vi "ANAL_SelectSpectrum.vi"(8 "Single Bin Selection":i32(slide) scale=1.0..58.0, 9 "Sweep Selection":i32(slide)=1 min=1 max=58 step=1 scale=1.0..58.0, 10 "Main Data Array":T1 {"Run Data Cluster"."Temperature B" scale=0.0..100.0; "Run Data Cluster"."Temperature A" scale=0.0..100.0}) -> (0 "Selected Spectrum":i32[](array[numeric]), 2 "Main Data Array Out":T1 {"Run Data Cluster"."Temperature B" scale=0.0..100.0; "Run Data Cluster"."Temperature A" scale=0.0..100.0})   [LabVIEW 2021]
uses:
  ANAL_Data.ctl
  XML_Cluster.ctl
  DAT_Cluster.ctl
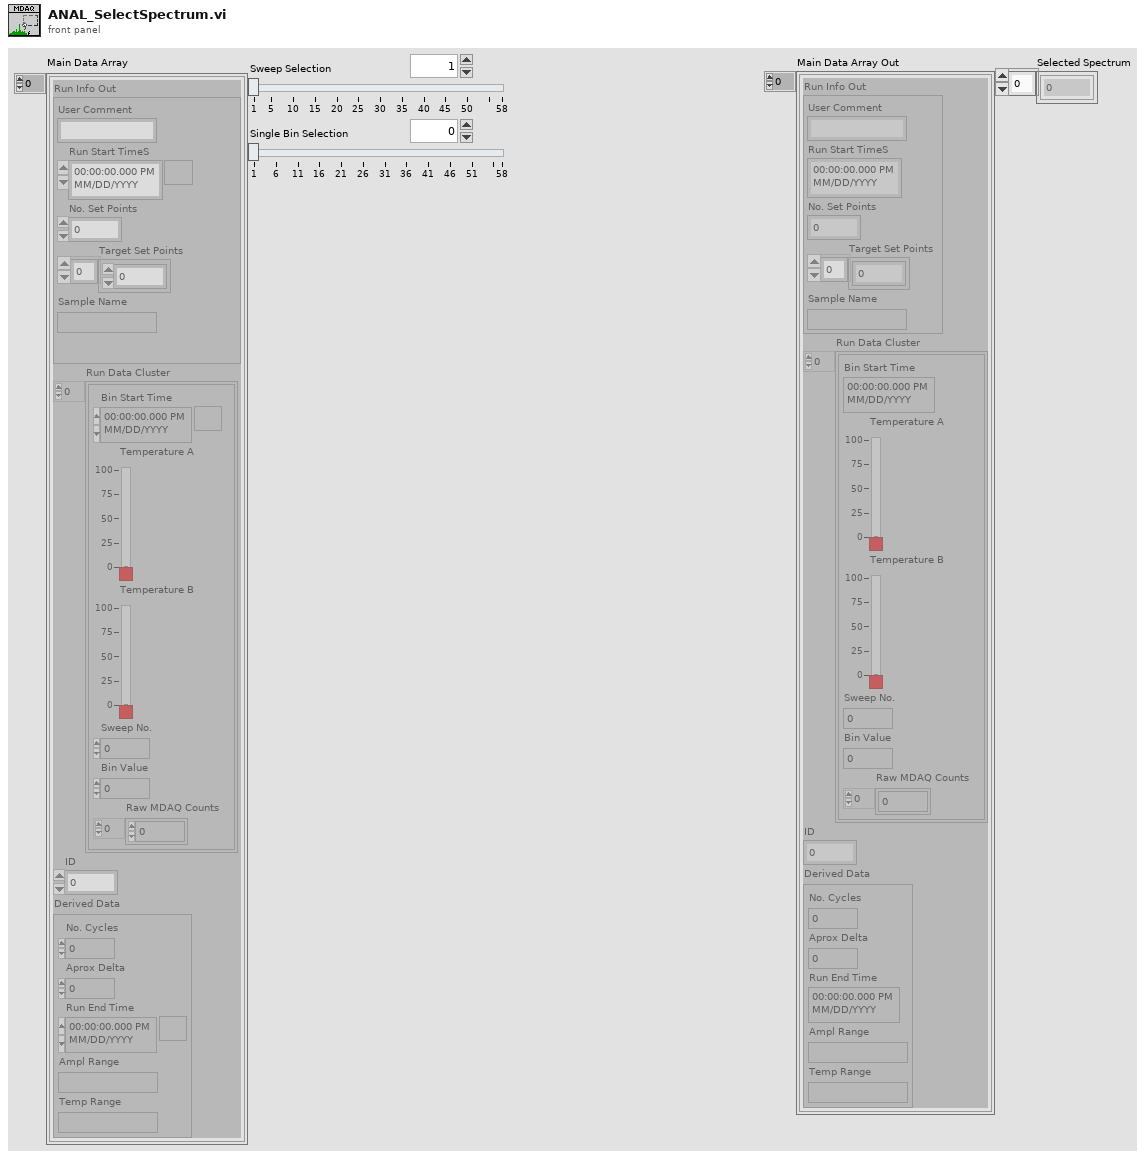
[diagram p1: front panel]
types:
  T1 = typedef "ANAL_Data.ctl" = cluster{"Run Info Out":T2, "Run Data Cluster":T3, "ID":u32, "Derived Data":cluster{"No. Cycles":u32, "Aprox Delta":dbl, "Run End Time":timestamp, "Ampl Range":string, "Temp Range":string}}[]
  T2 = typedef "XML_Cluster.ctl" = cluster{"User Comment":string, "Run Start TimeS":timestamp, "No. Set Points":u32, "Target Set Points":i32[], "Sample Name":string}
  T3 = typedef "DAT_Cluster.ctl" = cluster{"Bin Start Time":timestamp, "Temperature A":dbl, "Temperature B":dbl, "Sweep No.":i32, "Bin Value":i32, "Raw MDAQ Counts":i32[]}[]
  T4 = cluster{"Run Info Out":T2, "Run Data Cluster":T3, "ID":u32, "Derived Data":cluster{"No. Cycles":u32, "Aprox Delta":dbl, "Run End Time":timestamp, "Ampl Range":string, "Temp Range":string}}
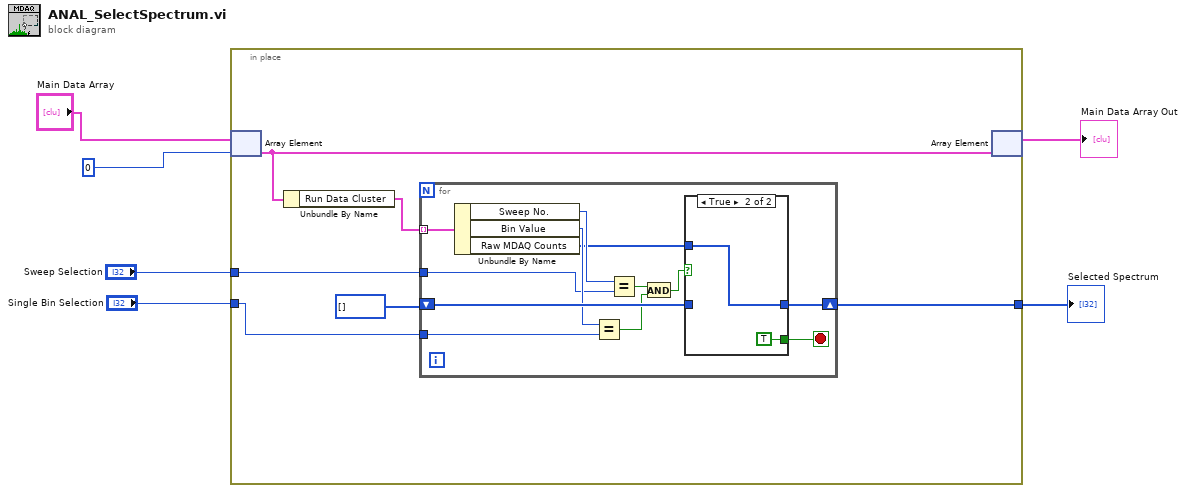
[diagram p0: block diagram]
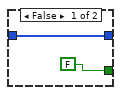
[diagram p2: hidden frame]
diagram:
  n1 = in-place {
    in-place-border: "Sweep Selection" -> [w9]
    in-place-border: "Single Bin Selection" -> [w8]
    in-place-border: [w7] -> w1
    n2 = in-place-array #1("Main Data Array", 0) -> (w12:T4)
    n3 = Unbundle By Name(w12) -> ("Run Data Cluster"=w11:T3)
    n4 = for {
      tunnel: w11 -> [w24] mode=indexing
      shift-right: [w22] -> w7
      shift-left: i32[] [] -> [w23]
      tunnel: w9 -> [w16]
      tunnel: w8 -> [w15]
      stop <- w13 stop-if-true
      n5 = Unbundle By Name(w24) -> ("Sweep No."=w18:i32, "Bin Value"=w17:i32, "Raw MDAQ Counts"=w14:i32[])
      n6 = Equal?(x=w17, y=w15) -> (x = y?=w19:bool)
      n7 = Equal?(x=w18, y=w16) -> (x = y?=w20:bool)
      n8 = And(x=w20, y=w19) -> (x .and. y?=w21:bool)
      n9 = case shown="True" w21 {
        tunnel: w23 -> [w26 _]
        tunnel: [w26 w28] -> w22
        tunnel: w14 -> [_ w28]
        tunnel: [FALSE TRUE] -> w13
        frame False {
        }
        frame True {
        }
      }
    }
    n10 = in-place-array #1(w12) -> (→"Main Data Array Out":T1)  [unwired: 1 out]
  }
  "Selected Spectrum" <- w1
